vi "setConnected.vi"(8 "error in (no error)":errorcluster, 9 "reason":i32, 10 "connected":bool, 11 "Connection in":refnum<class "Connection.lvclass">) -> (0 "error out":errorcluster, 3 "Connection out":refnum<class "Connection.lvclass">)   [LabVIEW 2013, in "Connection_GOSPL.lvlib" / "Connection.lvclass"]
uses:
  Connection.lvclass
  Connection.lvclass/Connection.ctl
  connection event -- cluster.ctl
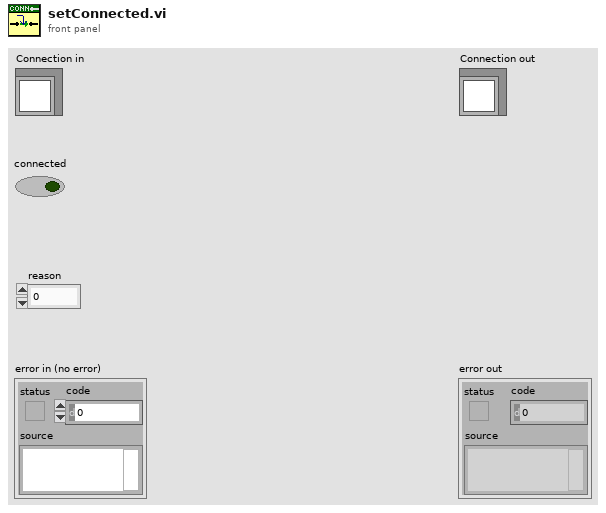
[diagram p1: front panel]
types:
  T1 = typedef "Connection_GOSPL.lvlib/Connection.lvclass/connection event -- cluster.ctl" = cluster{"connected":bool, "reason":i32}
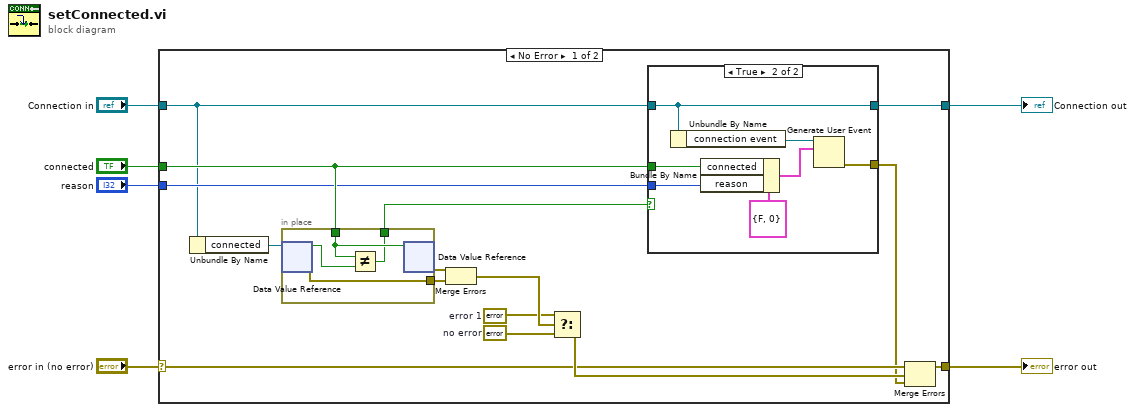
[diagram p0: block diagram]
diagram:
  n1 = case shown="No Error" "error in (no error)" {
    selector: "error in (no error)" -> [w14 w34]
    tunnel: [w20 w34] -> w6
    tunnel: "Connection in" -> [w10 w35]
    tunnel: "connected" -> [w12 _]
    tunnel: [w9 w35] -> w4
    tunnel: "reason" -> [w11 _]
    frame No Error {
      w7 = errorcluster {"status"=TRUE, "code"=1, "source"="Connection_GOSPL.lvlib:Connection.lvclass:setConnected.vi<APPEND>\n\n<b>Complete call chain:</b>\r\n     Connection_GOSPL.lvlib:Connection.lvclass:setConnected.vi"}  # error 1
      w18 = errorcluster {"status"=FALSE, "code"=0, "source"=""}  # no error
      n2 = Unbundle By Name(w10) -> ("connected"=w21:refnum<data-value>)
      n3 = in-place {
        in-place-border: w12 -> [w32]
        in-place-border: [w33] -> w17
        in-place-border: [w30] -> w13
        n4 = in-place-dvr #1(w21) -> (w31:bool, w33:errorcluster)
        n5 = Not Equal?(x=w32, y=w31) -> (x != y?=w30:bool)
        n6 = in-place-dvr #1(w32) -> (w16:errorcluster)  [unwired: 1 out]
      }
      n7 = Merge Errors(w16, w17) -> (w19:errorcluster)
      n8 = Select(t=w7, s=w19, f=w18) -> (s? t:f=w15:errorcluster)
      n9 = case shown="True" w13 {
        tunnel: w12 -> [_ w26]
        tunnel: w11 -> [_ w25]
        tunnel: w10 -> [w22 w29]
        tunnel: [w22 w29] -> w9
        tunnel: [_ w23] -> w8
        frame False {
        }
        frame True {
          n10 = Unbundle By Name(w29) -> ("connection event"=w28:refnum<user-event>)
          n11 = Bundle By Name(cluster=T1 {"connected"=FALSE, "reason"=0} ("Connection event"), "connected"=w26, "reason"=w25) -> (w24:T1)
          n12 = Generate User Event(user event=w28, event data cluster=w24) -> (error out=w23:errorcluster)  [unwired: 2 in, 1 out]
        }
      }
      n13 = Merge Errors(w14, w15, w8) -> (w20:errorcluster)
    }
    frame Error {
    }
  }
  "error out" <- w6
  "Connection out" <- w4
